vi "02 - 3rd Party Drivers.vi"   [LabVIEW 2021]
uses:
  <instrlib>/Agilent 34401/Public/VI Tree.vi
  <instrlib>/Agilent 34401/Agilent 34401.lvlib
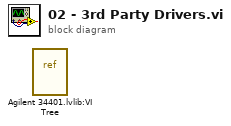
[diagram p0: block diagram]
diagram:
  n1 = vi-ref "Agilent 34401.lvlib:VI Tree.vi"() -> ()  [unwired: 1 out]
